vi "Get Provided Interface and Service Class.vi"(8 "error in":errorcluster, 11 "session factory in":refnum<class "Session Factory.lvclass">) -> (0 "error out":errorcluster, 1 "service class":string, 2 "provided interface":string, 3 "session factory out":refnum<class "Session Factory.lvclass">)   [LabVIEW 2020, in "NI Session Management niScope.lvlib" / "Session Factory.lvclass"]
uses:
  Session Factory.lvclass
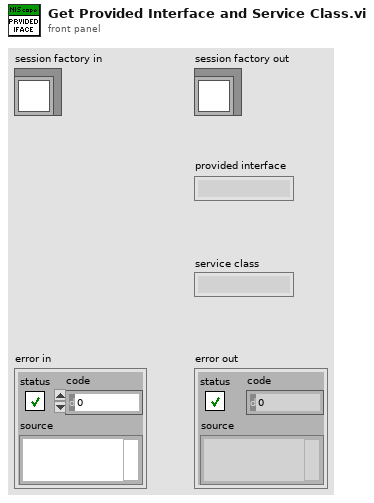
[diagram p1: front panel]
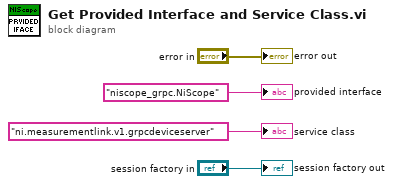
[diagram p0: block diagram]
diagram:
  "error out" <- "error in"
  "session factory out" <- "session factory in"
  "provided interface" <- "niscope_grpc.NiScope" ("provided interface")
  "service class" <- "ni.measurementlink.v1.grpcdeviceserver" ("service_class")
